vi "PassCmd.vi"(2 "超时毫秒(-1)":i32, 3 "cmd in":string, 4 "list ref":refnum<queue>) -> (0 "str out":string, 1 "cmd out":T1)   [LabVIEW 2012]
panel:
  out "new":bool
  in  "Msg":T2
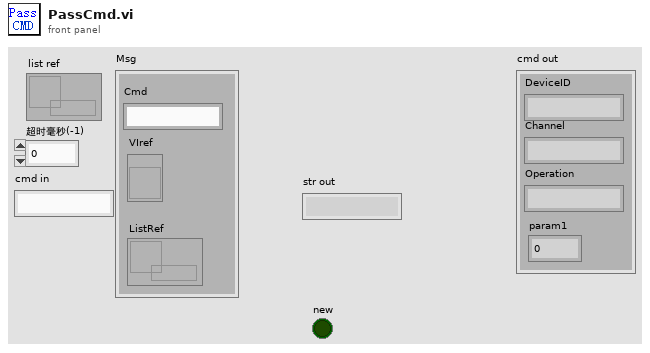
[diagram p1: front panel]
types:
  T1 = cluster{"DeviceID":string, "Channel":string, "param1":dbl, "Operation":string}
  T2 = cluster{"Cmd":string, "VIref":refnum<vi>, "ListRef":refnum<queue>}
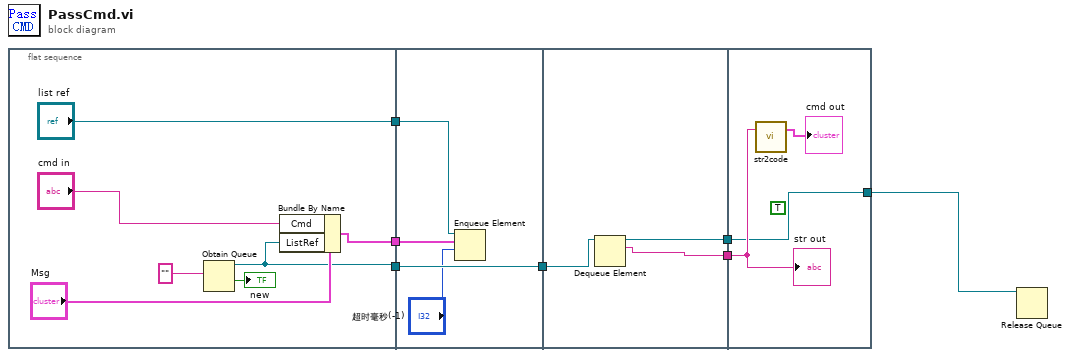
[diagram p0: block diagram]
diagram:
  n1 = flat-sequence {
    tunnel: ["list ref"] -> w7
    tunnel: [w10] -> w6
    tunnel: [w9] -> w5
    tunnel: w7 -> [w18]
    tunnel: w6 -> [w17]
    tunnel: w5 -> [w16]
    tunnel: [w16] -> w4
    tunnel: w4 -> [w21]
    tunnel: [w20] -> w3
    tunnel: [w19] -> w2
    tunnel: w3 -> [w24]
    tunnel: w2 -> [w22]
    tunnel: [w22] -> w1
    frame #0 {
      n2 = Obtain Queue(element data type="") -> (queue out=w9:refnum<queue>, created new?=→"new":bool)  [unwired: 4 in, 1 out]
      n3 = Bundle By Name(cluster="Msg", "Cmd"="cmd in", "ListRef"=w9) -> (w10:T2)
    }
    frame #1 {
      n4 = Enqueue Element(queue=w18, element=w17, timeout in ms (-1)="超时毫秒(-1)") -> ()  [unwired: 1 in, 3 out]
    }
    frame #2 {
      n5 = Dequeue Element(queue=w21) -> (queue out=w19:refnum<queue>, element=w20:string)  [unwired: 2 in, 2 out]
    }
    frame #3 {
      (unwired) TRUE ("强制销毁？(F)")
      n6 = call "str2code.vi"("input"=w24) -> ("Output"=→"cmd out":T1)  [unwired: 1 in, 1 out]
      "str out" <- w24
    }
  }
  n7 = Release Queue(queue=w1) -> ()  [unwired: 2 in, 3 out]
